vi "Test Startup Procedure.vi"(7 "Resistivity":T1, 8 "error in (no error)":errorcluster, 10 "Voltage Limit":dbl=2.0, 11 "Current Level":dbl=0.001) -> (0 "error out":errorcluster)   [LabVIEW 2016, in "Hall Effect Library.lvlib"]
doc: "This VI prepares the Hall Effect system's instruments for the Van Der Pauw and Hall Effect tests."
uses:
  Hall Effect Library.lvlib
  Public/Controls/Resisitivity.ctl
  Public/Controls/Switches.ctl
  Public/Controls/Voltmeters.ctl
  Global Variables/Instrument Locations.vi
  Global Variables/Instruments.vi
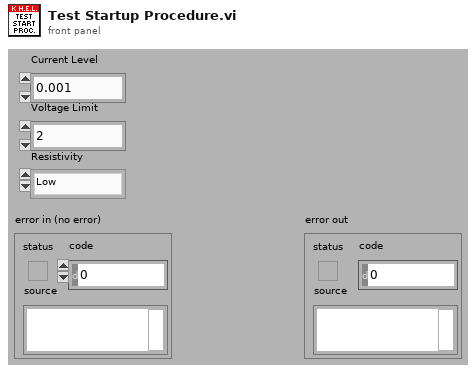
[diagram p1: front panel]
types:
  T1 = typedef "Hall Effect Library.lvlib/Resisitivity.ctl" = enum16{"Low", "High"}
  T2 = typedef "Hall Effect Library.lvlib/Voltmeters.ctl" = enum16{"2000", "2182A", "3706A"}
  T3 = typedef "Hall Effect Library.lvlib/Switches.ctl" = enum16{"3706A"}
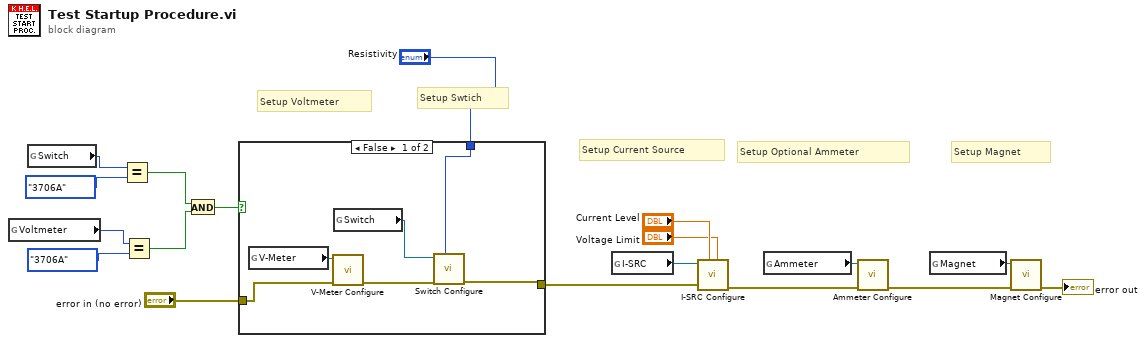
[diagram p0: block diagram]
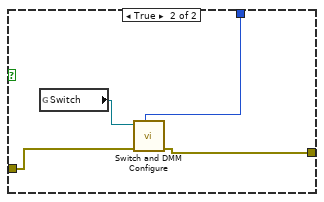
[diagram p2: hidden frame]
diagram:
  # "Setup Magnet"
  # "Setup Optional Ammeter"
  # "Setup Swtich"
  # "Setup Current Source"
  # "Setup Voltmeter"
  n1 = global read "Instruments.vi" "Voltmeter"() -> (w8:T2)
  n2 = global read "Instruments.vi" "Switch"() -> (w10:T3)
  n3 = Equal?(x=w10, y=Switches."3706A" ("Switch")) -> (x = y?=w6:bool)
  n4 = Equal?(x=w8, y=Voltmeters."3706A" ("Voltmeter")) -> (x = y?=w5:bool)
  n5 = And(x=w6, y=w5) -> (x .and. y?=w4:bool)
  n6 = case shown="False" w4 {
    tunnel: "error in (no error)" -> [w23 w28]
    tunnel: [w20 w27] -> w2
    tunnel: "Resistivity" -> [w19 w25]
    frame False {
      n7 = global read "Instrument Locations.vi" "V-Meter"() -> (w24:refnum<visa-resource-name>)
      n8 = call "V-Meter Configure.vi"("error in (no error)"=w23, "VISA resource name in"=w24) -> ("error out"=w21:errorcluster)  [unwired: 9 out]
      n9 = global read "Instrument Locations.vi" "Switch"() -> (w22:refnum<visa-resource-name>)
      n10 = call "Switch Configure.vi"("Resistivity"=w19, "error in (no error)"=w21, "VISA resource name in"=w22) -> ("error out"=w20:errorcluster)  [unwired: 8 out]
    }
    frame True {
      n11 = global read "Instrument Locations.vi" "Switch"() -> (w26:refnum<visa-resource-name>)
      n12 = call "Switch and DMM Configure.vi"("Resistivity"=w25, "error in (no error)"=w28, "VISA resource name"=w26) -> ("error out"=w27:errorcluster)  [unwired: 7 in, 1 out]
    }
  }
  n13 = global read "Instrument Locations.vi" "I-SRC"() -> (w16:refnum<visa-resource-name>)
  n14 = call "I-SRC Configure.vi"("Voltage Limit"="Voltage Limit", "Current Level"="Current Level", "error in (no error)"=w2, "VISA resource name in"=w16) -> ("error out"=w14:errorcluster)  [unwired: 2 in, 5 out]
  n15 = global read "Instrument Locations.vi" "Ammeter"() -> (w15:refnum<visa-resource-name>)
  n16 = call "Ammeter Configure.vi"("error in (no error)"=w14, "VISA resource name in"=w15) -> ("error out"=w11:errorcluster)  [unwired: 9 out]
  n17 = global read "Instrument Locations.vi" "Magnet"() -> (w12:refnum<visa-resource-name>)
  n18 = call "Magnet Configure.vi"("error in (no error)"=w11, "VISA resource name in"=w12) -> ("error out"=→"error out":errorcluster)  [unwired: 9 out]
